vi "SSI.vi"(6 "Command":T2, 8 "error in (no error)":errorcluster, 9 "Initialization Parameters":T1, 10 "Command args":string[](array[string]), 11 "Command name":string) -> (0 "error out":errorcluster, 3 "return arguments":string[](array[string]))   [LabVIEW 2020]
uses:
  typedefs/SSI_commands.ctl
  typedefs/SSI_Init_Params.ctl
panel:
  out "Response string":string
  out "Request string":string
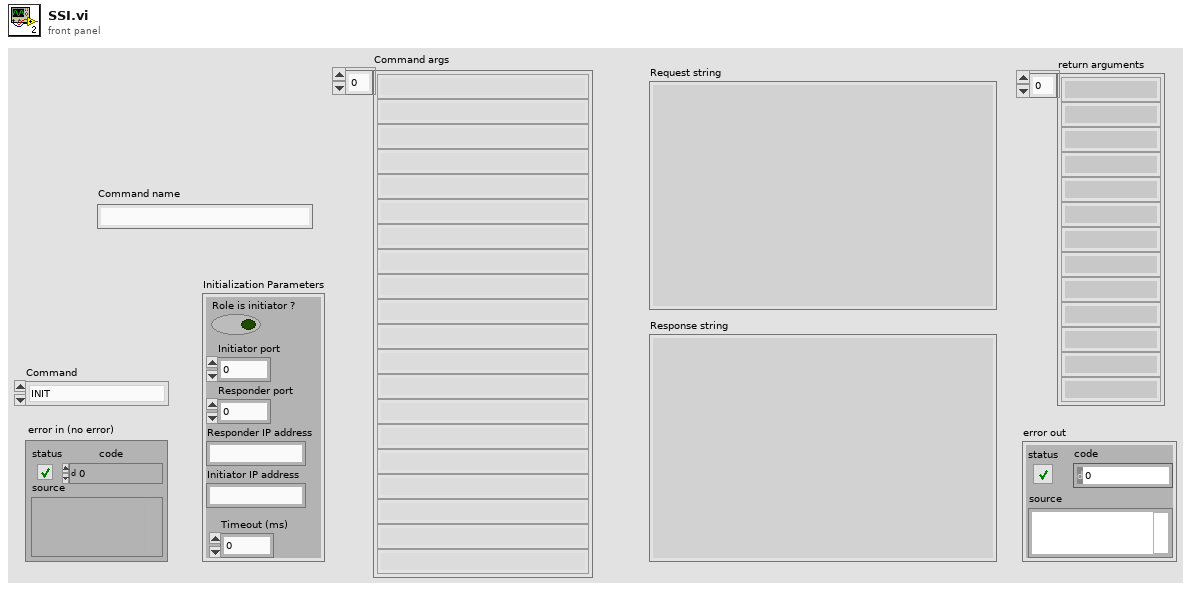
[diagram p1: front panel]
types:
  T1 = typedef "SSI_Init_Params.ctl" = cluster{"Role is initiator ?":bool, "Initiator port":i32, "Responder port":i32, "Responder IP address":string, "Initiator IP address":string, "Timeout (ms)":i32}
  T2 = typedef "SSI_commands.ctl" = enum16{"INIT", "ADD_COMMAND", "REMOVE_COMMAND", "QUERY", "SERVE"}
  T3 = enum16{"Standard", "Buffered", "CRLF", "Immediate"}
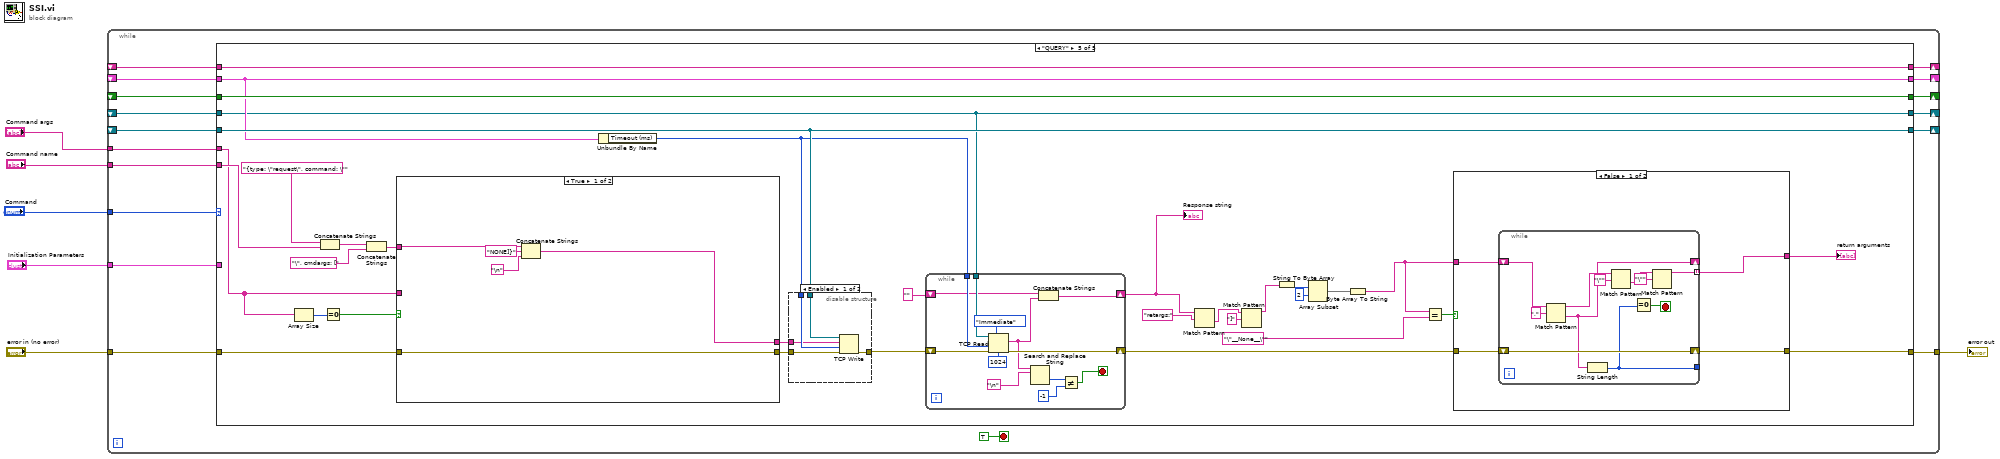
[diagram p0: block diagram]
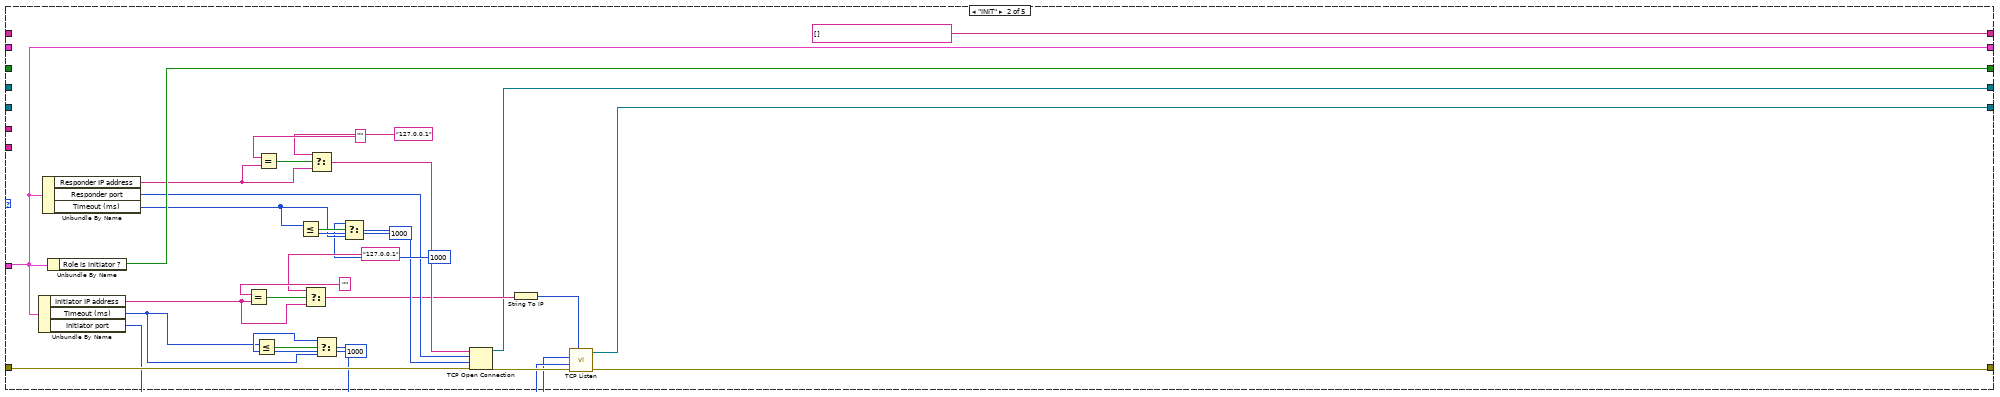
[diagram p3: hidden frame]
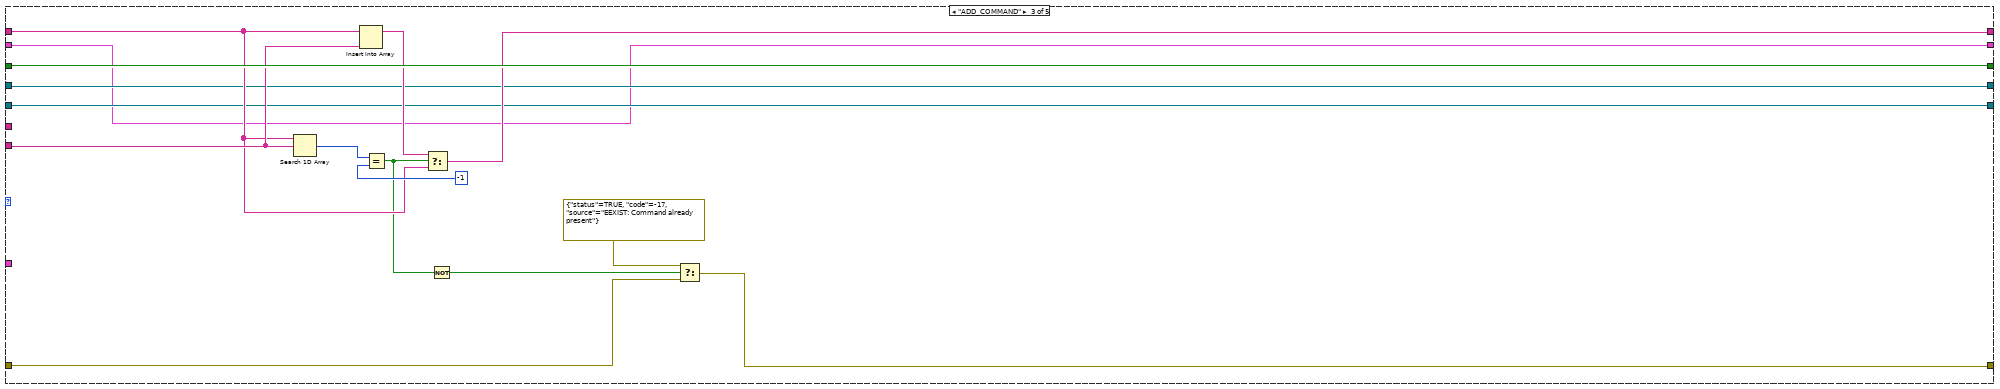
[diagram p4: hidden frame]
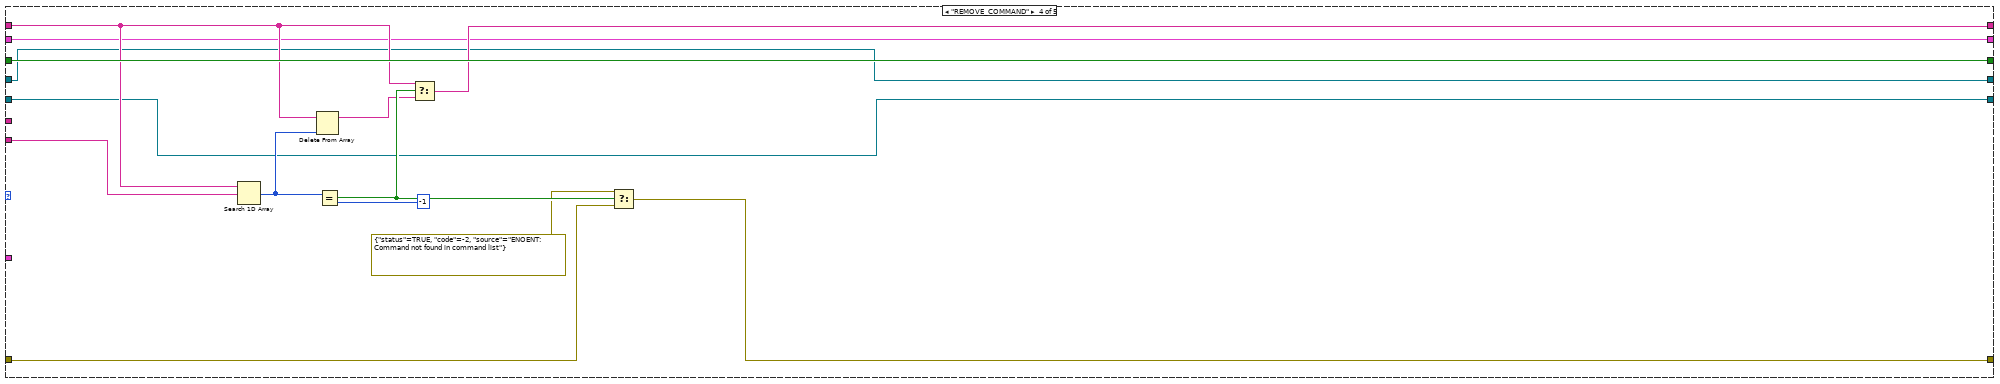
[diagram p5: hidden frame]
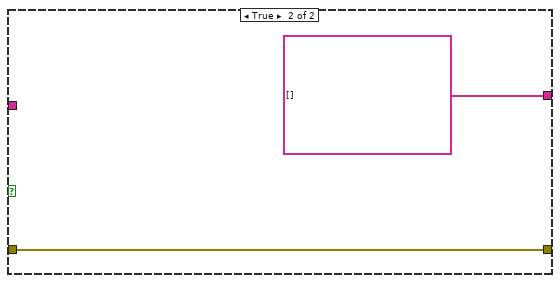
[diagram p6: hidden frame]
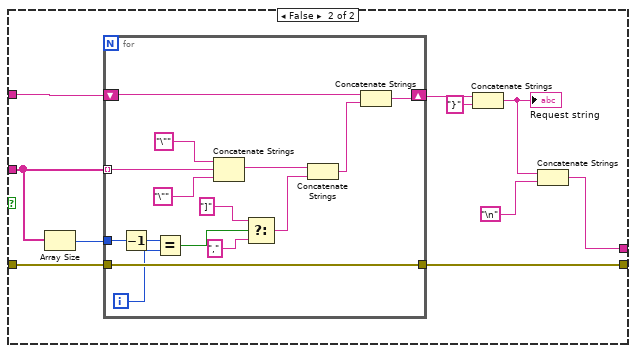
[diagram p7: hidden frame]
diagram:
  n1 = while {
    tunnel: "Command" -> [w22]
    tunnel: "error in (no error)" -> [w21]
    tunnel: [w20] -> w4
    shift-right: [w19] -> _
    shift-left: _ -> [w18]
    tunnel: "Command name" -> [w17]
    tunnel: "Command args" -> [w16]
    shift-right: [w15] -> _
    shift-left: _ -> [w14]
    tunnel: "Initialization Parameters" -> [w13]
    shift-right: [w12] -> _
    shift-left: _ -> [w10]
    shift-right: [w11] -> _
    shift-left: _ -> [w9]
    shift-right: [w8] -> _
    shift-left: _ -> [w7]
    stop <- TRUE stop-if-true
    n2 = case shown="\"QUERY\"" w22 {
      tunnel: w21 -> [w29 w58 w64 w80 w113]
      tunnel: [w29 w33 w63 w78 w97] -> w20
      tunnel: [w28 w57 w74 w88 w120] -> w19
      tunnel: w18 -> [w28 _ w74 w88 w120]
      tunnel: w17 -> [_ _ w71 w87 w116]
      tunnel: w16 -> [_ _ _ _ w105]
      tunnel: [w27 string[] [] w68 w81 w121] -> w15
      tunnel: w14 -> [w27 _ w69 w83 w121]
      tunnel: w13 -> [_ w30 _ _ _]
      tunnel: [w26 w32 w62 w77 w109] -> w12
      tunnel: [w25 w31 w61 w76 w119] -> w11
      tunnel: w10 -> [w26 _ w62 w77 w109]
      tunnel: w9 -> [w25 _ w61 w76 w119]
      tunnel: [w24 w30 w60 w75 w118] -> w8
      tunnel: w7 -> [w24 _ w60 w75 w118]
      frame Default {
      }
      frame "INIT" {
        w38 = 1000 ("y")
        n3 = Unbundle By Name(w30) -> ("Initiator IP address"=w54:string, "Timeout (ms)"=w37:i32, "Initiator port"=w35:i32)
        n4 = Unbundle By Name(w30) -> ("Responder IP address"=w49:string, "Responder port"=w42:i32, "Timeout (ms)"=w45:i32)
        n5 = Unbundle By Name(w30) -> ("Role is initiator ?"=w57:bool)
        n6 = Equal?(x="", y=w54) -> (x = y?=w55:bool)
        n7 = Less Or Equal?(x=w37, y=w38) -> (x <= y?=w39:bool)
        n8 = Equal?(x="", y=w49) -> (x = y?=w51:bool)
        n9 = Less Or Equal?(x=w45, y=1000) -> (x <= y?=w46:bool)
        n10 = Select(t="127.0.0.1", s=w55, f=w54) -> (s? t:f=w41:string)
        n11 = Select(t="127.0.0.1", s=w51, f=w49) -> (s? t:f=w48:string)
        n12 = Select(t=w38, s=w39, f=w37) -> (s? t:f=w36:i32)
        n13 = Select(t=1000, s=w46, f=w45) -> (s? t:f=w43:i32)
        n14 = TCP Open Connection(address=w48, remote port or service name=w42, timeout ms (60000)=w43, error in (no error)=w58) -> (connection ID=w32:refnum<k5>, error out=w40:errorcluster)  [unwired: 1 in]
        n15 = String To IP(1:w41) -> (0:w34:u32)
        n16 = call <vilib>:"TCP Listen.vi"("net address"=w34, "error in (no error)"=w40, "timeout ms (wait forever: -1)"=w36, "port"=w35) -> ("error out"=w33:errorcluster, "connection ID"=w31:refnum<k5>)  [unwired: 3 in, 3 out]
      }
      frame "ADD_COMMAND" {
        n17 = Search 1D Array(1D array=w69, element=w71) -> (index of element=w73:i32)  [unwired: 1 in]
        n18 = Insert Into Array(array=w69, new element=w71) -> (w70:string[])  [unwired: 1 in]
        n19 = Equal?(x=w73, y=-1) -> (x = y?=w67:bool)
        n20 = Select(t=w70, s=w67, f=w69) -> (s? t:f=w68:string[])
        n21 = Not(x=w67) -> (.not. x?=w66:bool)
        n22 = Select(t=errorcluster {"status"=TRUE, "code"=-17, "source"="EEXIST: Command already present"} ("error constant"), s=w66, f=w64) -> (s? t:f=w63:errorcluster)
      }
      frame "REMOVE_COMMAND" {
        n23 = Search 1D Array(1D array=w83, element=w87) -> (index of element=w86:i32)  [unwired: 1 in]
        n24 = Delete From Array(array=w83, index=w86) -> (array with subset deleted=w82:string[])  [unwired: 1 in, 1 out]
        n25 = Equal?(x=w86, y=-1) -> (x = y?=w84:bool)
        n26 = Select(t=w83, s=w84, f=w82) -> (s? t:f=w81:string[])
        n27 = Select(t=errorcluster {"status"=TRUE, "code"=-2, "source"="ENOENT: Command not found in command list"}, s=w84, f=w80) -> (s? t:f=w78:errorcluster)
      }
      frame "QUERY" {
        n28 = Array Size(array=w105) -> (size(s)=w104:i32)
        n29 = Concatenate Strings("{type: \"request\", command: \"" ("string"), w116) -> (w115:string)
        n30 = Equal To 0?(x=w104) -> (x = 0?=w103:bool)
        n31 = Concatenate Strings(w115, "\", cmdargs: [" ("string")) -> (w111:string)
        n32 = case shown="True" w103 {
          tunnel: w113 -> [w139 w153]
          tunnel: [w139 w152] -> w112
          tunnel: w111 -> [w143 w151]
          tunnel: [w140 w145] -> w108
          tunnel: w105 -> [_ w144]
          frame True {
            n33 = Concatenate Strings(w143, "NONE]}" ("string"), "\n") -> (w140:string)
          }
          frame False {
            n34 = Array Size(array=w144) -> (size(s)=w150:i32)
            n35 = for {
              tunnel: w153 -> [w168]
              tunnel: [w168] -> w152
              shift-right: [w154] -> w149
              shift-left: w151 -> [w156]
              tunnel: w144 -> [w167] mode=indexing
              tunnel: w150 -> [w163]
              i -> [w161]
              n36 = Decrement(x=w163) -> (x-1=w162:i32)
              n37 = Equal?(x=w162, y=w161) -> (x = y?=w160:bool)
              n38 = Concatenate Strings("\"" ("string"), w167, "\"" ("string")) -> (w164:string)
              n39 = Select(t="]", s=w160, f=",") -> (s? t:f=w157:string)
              n40 = Concatenate Strings(w164, w157) -> (w155:string)
              n41 = Concatenate Strings(w156, w155) -> (w154:string)
            }
            n42 = Concatenate Strings(w149, "}" ("string")) -> (w147:string)
            "Request string" <- w147
            n43 = Concatenate Strings(w147, "\n") -> (w145:string)
          }
        }
        n44 = Unbundle By Name(w118) -> ("Timeout (ms)"=w107:i32)
        n45 = disable-structure shown="Enabled" {
          disable-tunnel: w112 -> [w186 w187]
          disable-tunnel: [w185 w187] -> w110
          disable-tunnel: w119 -> [w184 _]
          disable-tunnel: w107 -> [w183 _]
          disable-tunnel: w108 -> [w182 _]
          frame Enabled {
            n46 = TCP Write(connection ID=w184, data in=w182, error in (no error)=w186, 9:w183) -> (error out=w185:errorcluster)  [unwired: 2 out]
          }
          frame Disabled {
          }
        }
        n47 = while {
          tunnel: w109 -> [w179]
          tunnel: w107 -> [w178]
          shift-right: [w180] -> w98
          shift-left: w110 -> [w181]
          shift-right: [w174] -> w102
          shift-left: "" -> [w175]
          stop <- w169 stop-if-true
          n48 = TCP Read(connection ID=w179, bytes to read=1024, error in (no error)=w181, 7:T3."Immediate" ("mode (standard)"), 9:w178) -> (data out=w173:string, error out=w180:errorcluster)  [unwired: 1 out]
          n49 = Search and Replace String(input string=w173, search string="\n") -> (offset past replacement=w171:i32)  [unwired: 6 in, 3 out]
          n50 = Concatenate Strings(w175, w173) -> (w174:string)
          n51 = Not Equal?(x=w171, y=-1) -> (x != y?=w169:bool)
        }
        "Response string" <- w102
        n52 = Match Pattern(string=w102, regular expression="retargs:" ("search string")) -> (after substring=w94:string)  [unwired: 1 in, 3 out]
        n53 = Match Pattern(string=w94, regular expression="]") -> (before substring=w93:string)  [unwired: 1 in, 3 out]
        n54 = String To Byte Array(string=w93) -> (unsigned byte array=w92:u8[])
        n55 = Array Subset(array=w92, index=2) -> (w90:u8[])  [unwired: 1 in]
        n56 = Byte Array To String(unsigned byte array=w90) -> (string=w89:string)
        n57 = Equal?(x=w89, y="\"__None__\"") -> (x = y?=w99:bool)
        n58 = case shown="False" w99 {
          tunnel: w98 -> [w125 w138]
          tunnel: [w123 w138] -> w97
          tunnel: [w122 string[] []] -> w96
          tunnel: w89 -> [w124 _]
          frame False {
            n59 = while {
              shift-right: [w134] -> w123
              shift-left: w125 -> [w134]
              shift-right: [w128] -> _
              shift-left: w124 -> [w136]
              tunnel: [w129] -> w122 mode=indexing
              tunnel: [w126] -> _
              stop <- w127 stop-if-true
              n60 = Match Pattern(string=w136, regular expression=",") -> (before substring=w133:string, after substring=w128:string)  [unwired: 1 in, 2 out]
              n61 = String Length(string=w128) -> (length=w126:i32)
              n62 = Match Pattern(string=w133, regular expression="\"") -> (after substring=w131:string)  [unwired: 1 in, 3 out]
              n63 = Equal To 0?(x=w126) -> (x = 0?=w127:bool)
              n64 = Match Pattern(string=w131, regular expression="\"") -> (before substring=w129:string)  [unwired: 1 in, 3 out]
            }
          }
          frame True {
          }
        }
        "return arguments" <- w96
      }
    }
  }
  "error out" <- w4
